vi "LVClass_HasoData equalize AB.vi"(0 "HasoData A in":refnum<class "HasoData.lvclass">, 5 "HasoData B in":refnum<class "HasoData.lvclass">, 11 "error in (no error)":errorcluster) -> (4 "HasoData A out (A = B)":refnum<class "HasoData.lvclass">, 6 "HasoData B (dup)":refnum<class "HasoData.lvclass">, 15 "error out":errorcluster)   [LabVIEW 2020, in "HasoData.lvclass"]
doc: "HasoData assignment.\n\n--------------------------------------------------------------------------------\n\n<B>HasoData_dstIn </B> : HasoData object destination.\n<B>HasoData_dstOut </B> : HasoData object destination.\n<B>HasoData_src </B> : HasoData object source.\n<B>ErrorIn </B> : Error\n<B>ErrorOut </B> : Error\n\n--------------------------------------------------------------------------------"
uses:
  HasoData.lvclass
  HasoData.lvclass/HasoData.ctl
  LVClass_HasoData Read HasoData - property.vi
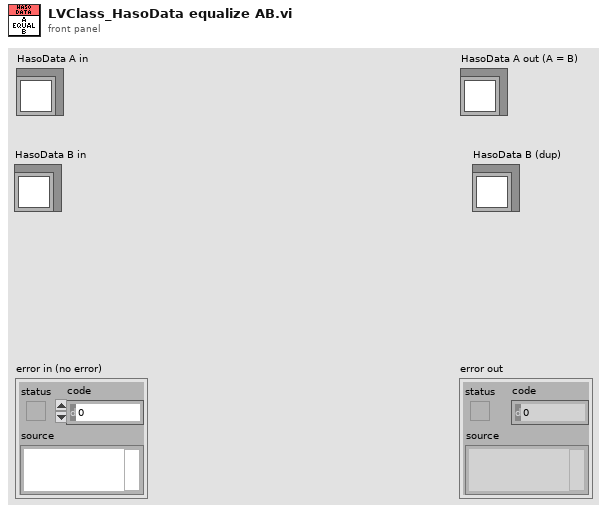
[diagram p1: front panel]
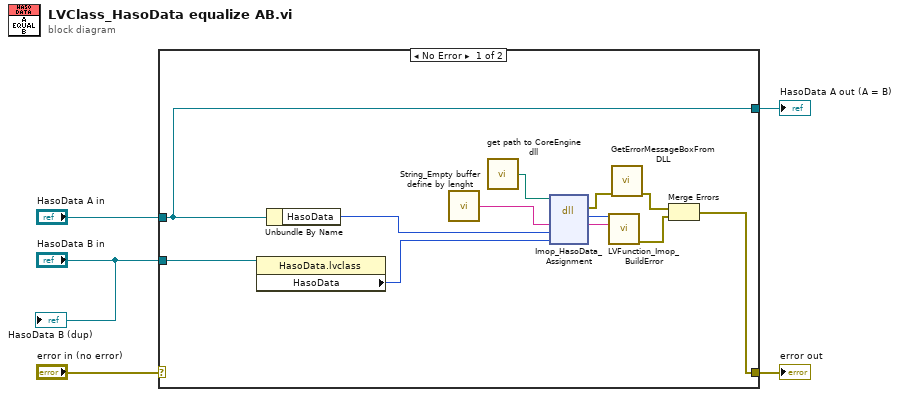
[diagram p0: block diagram]
diagram:
  n1 = case shown="No Error" "error in (no error)" {
    selector: "error in (no error)" -> [_ w19]
    tunnel: [w6 w19] -> w4
    tunnel: [w9 w18] -> w2
    tunnel: "HasoData A in" -> [w9 w18]
    tunnel: "HasoData B in" -> [w12 _]
    frame No Error {
      n2 = property class="HasoData.lvclass"(reference=w12) -> ("HasoData"=w11:i32)  [unwired: 1 in, 2 out]
      n3 = Unbundle By Name(w9) -> ("HasoData"=w10:i32)
      n4 = call "String_Empty buffer define by lenght.vi"() -> ("Empty buffer"=w15:string)  [unwired: 1 in]
      n5 = call "get path to CoreEngine dll.vi"() -> ("path to c_interface_vc100.dll"=w16:path)  [unwired: 12 in, 3 out]
      n6 = dll-call lib="D:/soft/HASO_v3/SVN_trunk/ImOpCoreEngine4_LV2011/DLLs/c_interface_vc100.dll" fn="Imop_HasoData_Assignment"(path in=w16, "message"=w15, "HasoDataA"=w10, "HasoDataB"=w11) -> (error out=w17:errorcluster, "return type"=w13:i32, "message"=w14:string)  [unwired: 4 in, 1 out]
      n7 = call "LVFunction_Imop_BuildError.vi"("code"=w13, "String to Prepend to source (\"\")"=w14) -> ("error out"=w7:errorcluster)  [unwired: 13 in]
      n8 = call "GetErrorMessageBoxFromDLL.vi"("error IN"=w17) -> ("error OUT"=w8:errorcluster)  [unwired: 10 in]
      n9 = Merge Errors(w8, w7) -> (w6:errorcluster)
    }
    frame Error {
    }
  }
  "error out" <- w4
  "HasoData A out (A = B)" <- w2
  "HasoData B (dup)" <- "HasoData B in"
